vi "Dequeue element.vi"(8 "error in (no error)":errorcluster) -> (0 "error out":errorcluster, 3 "Message":T1={"State"=enum."Init: Which Project?", "Data"=variant})   [LabVIEW 2018, in "Covers-o-meter.lvlib"]
doc: "Dequeues element"
uses:
  Covers-o-meter.lvlib
  ctl/Message--enum.ctl
  ctl/State--enum.ctl
  ctl/Queue action--enum.ctl
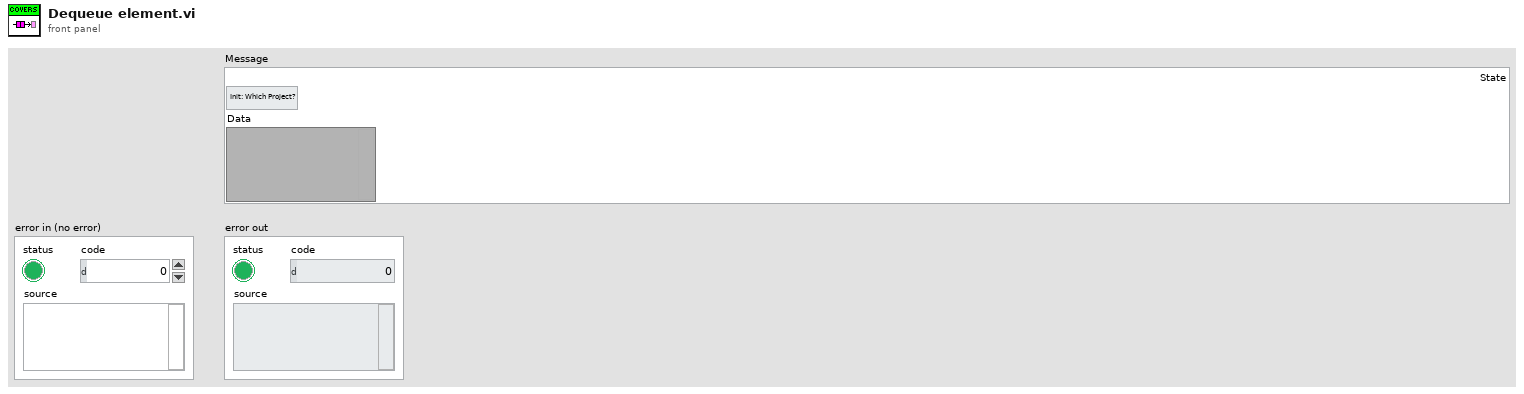
[diagram p1: front panel]
types:
  T1 = typedef "Covers-o-meter.lvlib/Message--enum.ctl" = cluster{"State":T2, "Data":variant}
  T2 = typedef "Covers-o-meter.lvlib/State--enum.ctl" = enum16{"Init", "Init: Read req tags", "Init Data: All Projects", "Init: Which Project?", "Update Requirements tags", "Get all project strings", "Search proj for tags", "Subroutine", "Update Project", "Start Button Pressed", "Start timer", "Error", "Close", "UI - Refresh Timer ", "UI - refresh graph", "UI - Refresh Tree"}
  T3 = typedef "Covers-o-meter.lvlib/Queue action--enum.ctl" = enum16{"Create", "Get", "Destroy"}
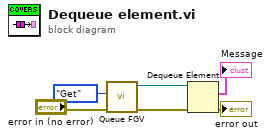
[diagram p0: block diagram]
diagram:
  n1 = call "Queue FGV.vi"("error in"="error in (no error)", "Queue Action"=Queue_action--enum."Get") -> ("error out"=w1:errorcluster, "Queue reference"=w2:refnum<queue>)  [unwired: 8 in]
  n2 = Dequeue Element(queue=w2, error in (no error)=w1) -> (element=→"Message":T1, error out=→"error out":errorcluster)  [unwired: 1 in, 2 out]
